vi "Execute.vi"() -> ()   [LabVIEW 2018]
uses:
  <vilib>/rvi/Emulation/niFpgaGetClockAttributes.vi
  <vilib>/rvi/Emulation/niFpgaSctlEmulationGetInTimedLoop.vi
  <vilib>/rvi/Emulation/niFpgaEmulationReportErrorSimple.vi
  <vilib>/rvi/DataTransferAndStorage/Container/Common/niFpgaContainerExecOnDevCompGetState.vi
  <vilib>/rvi/Emulation/niFpgaEmulationIsFPGAContextNoSignature.vi
  <vilib>/rvi/errors/niFpgaSetErrorForExecOnDevCompSimple.vi
  <vilib>/rvi/eio/common/nirviEmuReportErrorAndStop.vi
  <vilib>/rvi/DataTransferAndStorage/Container/Common/niFpgaContainerGetUniqueNameForEmu.vi
  <vilib>/rvi/FIFO/Fifo_Resource/nirvififoEmulationSetSize.vi
  <vilib>/rvi/FIFO/Fifo_Resource/nirviFifoEmulationQueueMgr.vi
  <instcachedir>/0/nirviFifoEmulationQueueMgr_E5CAEC123FF24DC58D834DCA3CDAA9B5.lvgen/nirviFifoEmulationQueueMgr_E5CAEC123FF24DC58D834DCA3CDAA9B5_001.vi
  <vilib>/rvi/FIFO/Fifo_Resource/nirvififoEmulationDetermineInputValidOut.vi
  <vilib>/rvi/FIFO/Fifo_Resource/nirvififoEmulationCreateLock.vi
  <vilib>/rvi/Emulation/niFpgaProcessEmulError.vi
  <vilib>/rvi/FIFO/Fifo_Resource/nirvififoEmulationObtainLock.vi
  <vilib>/rvi/FIFO/Fifo_Resource/nirvififoEmulationReleaseLock.vi
  <vilib>/rvi/occurrence/nirviWaitOnOccurrenceBase.vi
  <vilib>/rvi/errors/nirviReportUnexpectedCaseInternalError.vi
  <vilib>/rvi/errors/nirviReportUnexpectedCaseInternalError (U32).vi
  <vilib>/Utility/error.llb/Clear Errors.vi
  <vilib>/rvi/interface/RandomDataEmulation/niFpgaRandomDataHandleErrors.vi
  <vilib>/rvi/eio/common/nirviEmuTemplateMethod_errors.vi
  <vilib>/rvi/Emulation/niFpgaCriticalErrorInLSC.vi
  <vilib>/rvi/DataTransferAndStorage/Container/XNode/niFpgaContainer.xnode
  <vilib>/rvi/FIFO/Fifo_Resource/niFpgaFifoEmulationRefIn.vi
  <vilib>/eio/EIOMethodNode/EIOMethodNode.xnode
panel:
  in  "Instructions":u8[](array[numeric])=[0, 0, 0, 0, 0, 0, 0, 0, 0, 0, 0, 0, 0, 0, 0, 0, 0, 0, 0, 0, 0, 0, 0, 0, 0, 0, 0, 0, 0, 0, 0, 0, 0, 0, 0, 0, 0, 0, 0, 0, 0, 0, 0, 0, 0, 0, 0, 0, 0, 0, 0, 0, 0, 0, 0, 0, 0, 0, 0, 0, 0, 0, 0, 0, 0, 0, 0, 0, 0, 0, 0, 0, 0, 0, 0, 0, 0, 0, 0, 0, 0, 0, 0, 0, 0, 0, 0, 0, 0, 0, 0, 0, 0, 0, 0, 0, 0, 0, 0, 0]
  in  "IP":i16
  in  "DebugOut":refnum<k21>
  out "Output":u8[](array[numeric])
  in  "cRIO I/O Device":refnum<k21>
  in  "Command FIFO":refnum<k21>
  out "error out":errorcluster
  in  "error in (no error)":errorcluster
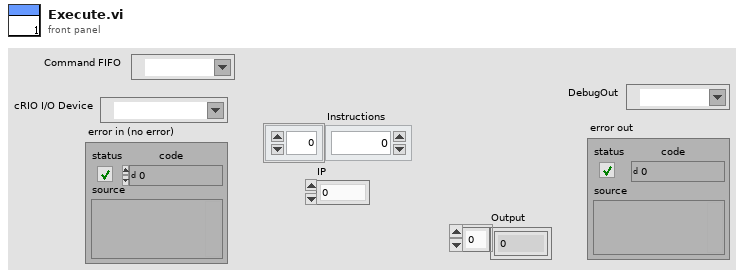
[diagram p1: front panel]
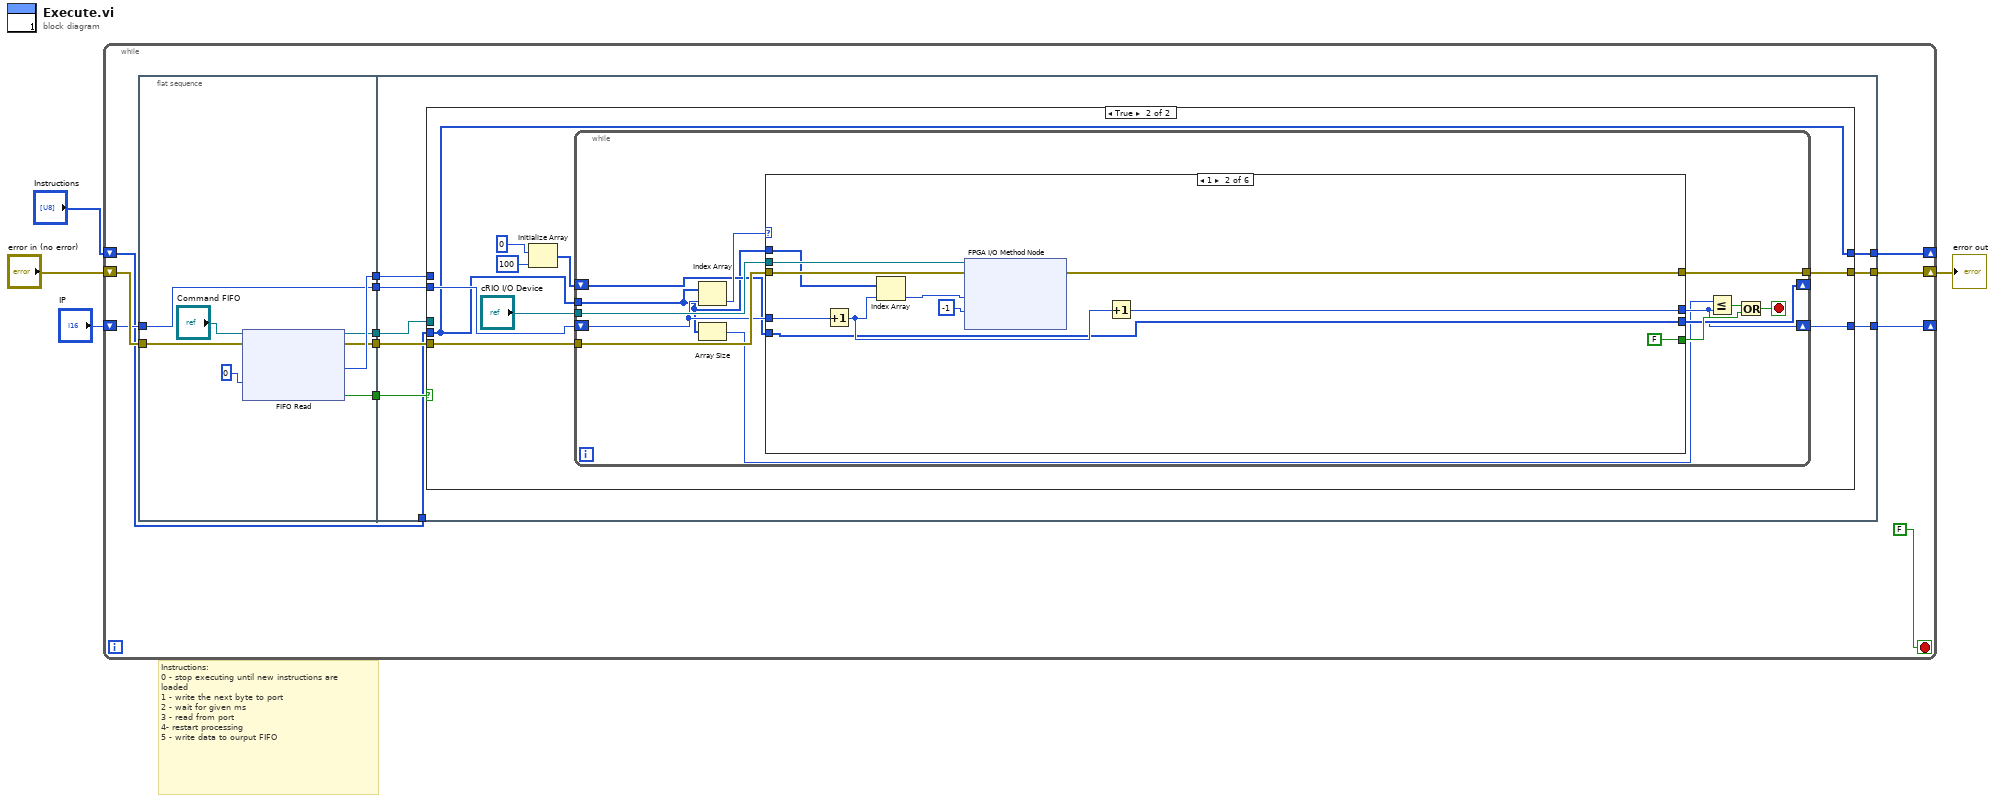
[diagram p0: block diagram]
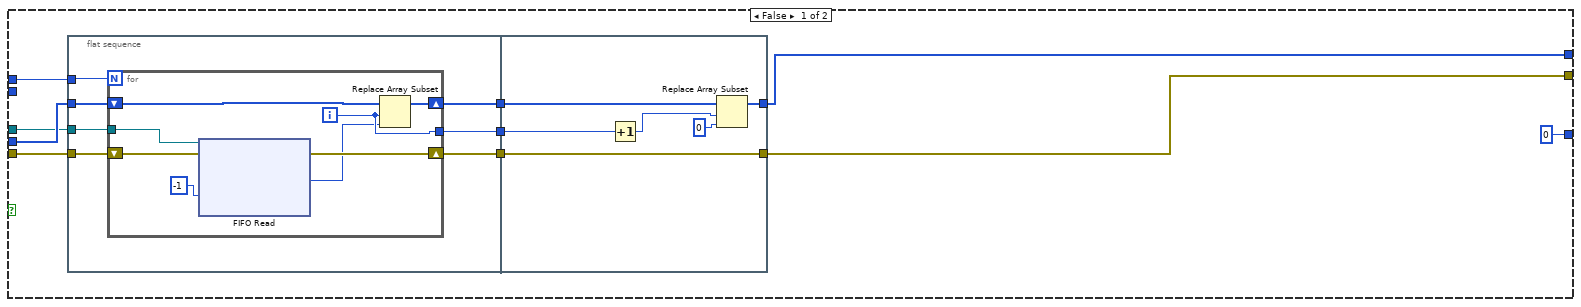
[diagram p2: hidden frame]
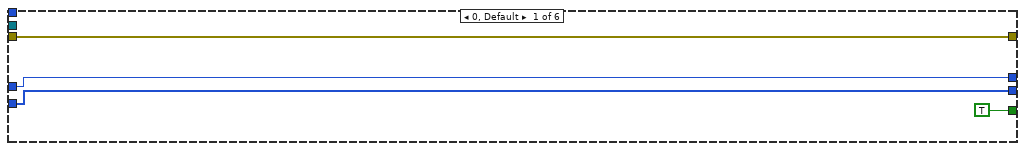
[diagram p3: hidden frame]
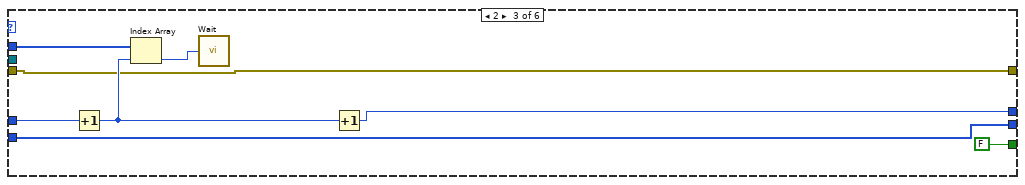
[diagram p4: hidden frame]
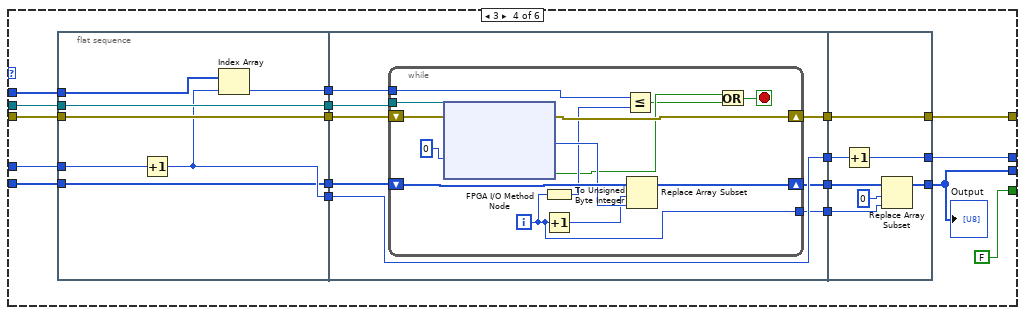
[diagram p5: hidden frame]
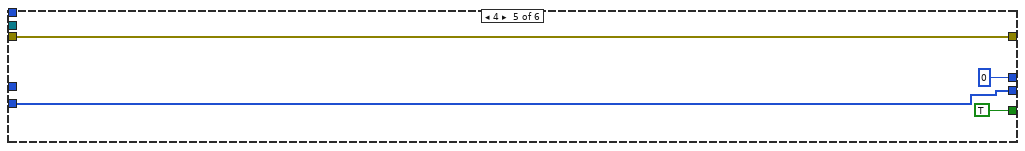
[diagram p6: hidden frame]
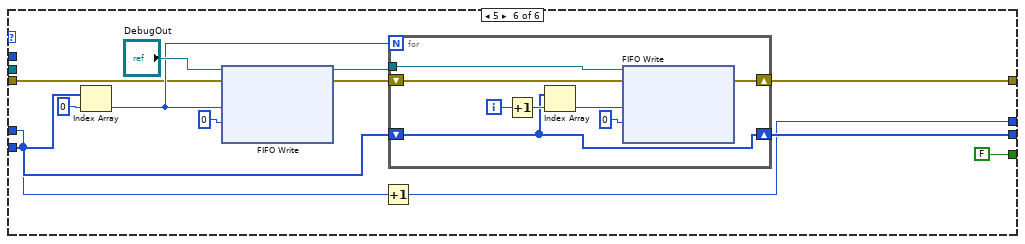
[diagram p7: hidden frame]
diagram:
  # "Instructions:\n0 - stop executing until new instructions are loaded\n1 - write the next byte to port\n2 - wait for given ms\n3 - read from port\n4- restart processing\n5 - write data to ourput FIFO"
  n1 = while {
    shift-right: [w7] -> w3
    shift-left: "error in (no error)" -> [w16]
    shift-right: [w8] -> _
    shift-left: "IP" -> [w10]
    shift-right: [w5] -> _
    shift-left: "Instructions" -> [w6]
    stop <- FALSE stop-if-true
    n2 = flat-sequence {
      tunnel: w16 -> [w24]
      tunnel: [w23] -> w15
      tunnel: [w22] -> w14
      tunnel: [w21] -> w13
      tunnel: [w19] -> w12
      tunnel: w10 -> [w17]
      tunnel: [w17] -> w9
      tunnel: w15 -> [w33]
      tunnel: w14 -> [w32]
      tunnel: w13 -> [w31]
      tunnel: w12 -> [w30]
      tunnel: w9 -> [w29]
      tunnel: [w28] -> w8
      tunnel: [w27] -> w7
      tunnel: w6 -> [w26]
      tunnel: [w25] -> w5
      frame #0 {
        n3 = xnode ("FIFO Read")("Timeout"=0, "error in (no error)"=w24, "FIFO In"="Command FIFO") -> ("Element"=w23:u8, "Timed Out?"=w22:bool, "error out"=w21:errorcluster, "FIFO Out"=w19:refnum<k21>)
      }
      frame #1 {
        n4 = case shown="True" w32 {
          tunnel: w31 -> [w43 w73]
          tunnel: w33 -> [w42 _]
          tunnel: w26 -> [w41 w65]
          tunnel: w30 -> [w37 _]
          tunnel: w29 -> [_ w71]
          tunnel: [i16 0 ("IP") w70] -> w28
          tunnel: [w35 w66] -> w27
          tunnel: [w34 w65] -> w25
          frame False {
            n5 = flat-sequence {
              tunnel: w41 -> [w47]
              tunnel: w42 -> [w48]
              tunnel: w43 -> [w50]
              tunnel: [w49] -> w40
              tunnel: [w46] -> w39
              tunnel: [w45] -> w38
              tunnel: w37 -> [w44]
              tunnel: [w64] -> w35
              tunnel: w40 -> [w64]
              tunnel: w39 -> [w63]
              tunnel: w38 -> [w62]
              tunnel: [w59] -> w34
              frame #0 {
                n6 = for {
                  N: w48 -> [_]
                  shift-right: [w57] -> w49
                  shift-left: w50 -> [w58]
                  shift-right: [w54] -> w46
                  shift-left: w47 -> [w56]
                  tunnel: [w53] -> w45
                  tunnel: w44 -> [w52]
                  i -> [w53]
                  n7 = xnode ("FIFO Read")("Timeout"=-1, "error in (no error)"=w58, "FIFO In"=w52) -> ("Element"=w51:u8, "error out"=w57:errorcluster)  [unwired: 2 out]
                  n8 = Replace Array Subset(array=w56, new element=w51, index=w53) -> (w54:u8[])
                }
              }
              frame #1 {
                n9 = Increment(x=w62) -> (x+1=w61:i32)
                n10 = Replace Array Subset(array=w63, new element=u8 0 ("new element/subarray"), index=w61) -> (w59:u8[])
              }
            }
          }
          frame True {
            n11 = Initialize Array(u8 0 ("element"), 100 ("dimension size")) -> (w67:u8[])
            n12 = while {
              tunnel: w65 -> [w79]
              tunnel: "cRIO I/O Device" -> [w85]
              tunnel: w73 -> [w84]
              shift-right: [w76] -> w70
              shift-left: w71 -> [w82]
              shift-right: [w80] -> _
              shift-left: w67 -> [w81]
              tunnel: [w74] -> w66
              stop <- w78 stop-if-true
              n13 = Index Array(array=w79, index=w82) -> (element=w83:u8)
              n14 = Array Size(array=w79) -> (size(s)=w75:i32)
              n15 = case shown="1" w83 {
                tunnel: [TRUE FALSE FALSE FALSE TRUE FALSE] -> w86
                tunnel: w85 -> [_ w99 _ w120 _ _]
                tunnel: w84 -> [w87 w100 w102 w121 w164 w170]
                tunnel: w82 -> [w89 w95 w107 w117 _ w175]
                tunnel: [w89 w93 w106 w126 i16 0 w174] -> w76
                tunnel: w79 -> [_ w97 w109 w127 _ _]
                tunnel: [w88 w92 w103 w113 w165 w177] -> w80
                tunnel: w81 -> [w88 w92 w103 w112 w165 w178]
                tunnel: [w87 w91 w102 w110 w164 w173] -> w74
                frame 0, Default {
                }
                frame 1 {
                  n16 = Increment(x=w95) -> (x+1=w94:i16)
                  n17 = Index Array(array=w97, index=w94) -> (element=w96:u8)
                  n18 = xnode "FPGA I/O Method Node"("error in"=w100, "FPGA I/O In"=w99, "Data"=w96, "Timeout (ms)"=-1) -> ("error out"=w91:errorcluster)  [unwired: 2 out]
                  n19 = Increment(x=w94) -> (x+1=w93:i16)
                }
                frame 2 {
                  n20 = Increment(x=w107) -> (x+1=w105:i16)
                  n21 = Index Array(array=w109, index=w105) -> (element=w108:u8)
                  n22 = call "Wait"("Count(mSec)"=w108) -> ()  [unwired: 1 out]
                  n23 = Increment(x=w105) -> (x+1=w106:i16)
                }
                frame 3 {
                  n24 = flat-sequence {
                    tunnel: w127 -> [w134]
                    tunnel: [w133] -> w123
                    tunnel: w121 -> [w132]
                    tunnel: [w132] -> w122
                    tunnel: w120 -> [w131]
                    tunnel: [w131] -> w119
                    tunnel: w117 -> [w130]
                    tunnel: [w129] -> w116
                    tunnel: w112 -> [w128]
                    tunnel: [w128] -> w111
                    tunnel: [w142] -> w125
                    tunnel: [w141] -> w124
                    tunnel: w123 -> [w137]
                    tunnel: w122 -> [w140]
                    tunnel: w119 -> [w139]
                    tunnel: [w138] -> w118
                    tunnel: w116 -> [w142]
                    tunnel: [w136] -> w114
                    tunnel: w111 -> [w135]
                    tunnel: [w162] -> w110
                    tunnel: [w161] -> w126
                    tunnel: w125 -> [w163]
                    tunnel: w124 -> [w162]
                    tunnel: w118 -> [w160]
                    tunnel: [w159] -> w113
                    tunnel: w114 -> [w158]
                    frame #0 {
                      n25 = Increment(x=w130) -> (x+1=w129:i16)
                      n26 = Index Array(array=w134, index=w129) -> (element=w133:u8)
                    }
                    frame #1 {
                      n27 = while {
                        shift-right: [w155] -> w141
                        shift-left: w140 -> [w156]
                        shift-right: [w154] -> w138
                        shift-left: w135 -> [w153]
                        tunnel: w139 -> [w152]
                        tunnel: w137 -> [w146]
                        tunnel: [w145] -> w136
                        i -> [w145]
                        stop <- w148 stop-if-true
                        n28 = xnode "FPGA I/O Method Node"("error in"=w156, "FPGA I/O In"=w152, "Timeout (ms)"=0) -> ("error out"=w155:errorcluster, "Data"=w151:u8, "Timed Out"=w144:bool)  [unwired: 1 out]
                        n29 = To Unsigned Byte Integer(number=w145) -> (unsigned 8bit integer=w147:u8)
                        n30 = Increment(x=w145) -> (x+1=w149:i32)
                        n31 = Less Or Equal?(x=w146, y=w147) -> (x <= y?=w143:bool)
                        n32 = Replace Array Subset(array=w153, new element=w151, index=w149) -> (w154:u8[])
                        n33 = Or(x=w144, y=w143) -> (x .or. y?=w148:bool)
                      }
                    }
                    frame #2 {
                      n34 = Increment(x=w163) -> (x+1=w161:i16)
                      n35 = Replace Array Subset(array=w160, new element=w158, index=0) -> (w159:u8[])
                    }
                  }
                  "Output" <- w113
                }
                frame 4 {
                }
                frame 5 {
                  n36 = Index Array(array=w178, index=0) -> (element=w171:u8)
                  n37 = xnode "FIFO Write"("Element"=w171, "Timeout"=0, "error in (no error)"=w170, "FIFO In"="DebugOut") -> ("error out"=w169:errorcluster, "FIFO Out"=w172:refnum<k21>)  [unwired: 1 out]
                  n38 = Increment(x=w175) -> (x+1=w174:i16)
                  n39 = for {
                    N: w171 -> [_]
                    shift-right: [w186] -> w177
                    shift-left: w178 -> [w186]
                    tunnel: w172 -> [w185]
                    shift-right: [w181] -> w173
                    shift-left: w169 -> [w184]
                    i -> [w188]
                    n40 = Increment(x=w188) -> (x+1=w187:i32)
                    n41 = Index Array(array=w186, index=w187) -> (element=w182:u8)
                    n42 = xnode "FIFO Write"("Element"=w182, "Timeout"=0, "error in (no error)"=w184, "FIFO In"=w185) -> ("error out"=w181:errorcluster)  [unwired: 2 out]
                  }
                }
              }
              n43 = Less Or Equal?(x=w75, y=w76) -> (x <= y?=w77:bool)
              n44 = Or(x=w77, y=w86) -> (x .or. y?=w78:bool)
            }
          }
        }
      }
    }
  }
  "error out" <- w3
